vi "Stop Core.vi"(10 "final error code":i32, 11 "CONTADOR_CON_LIMITES in":refnum<class "CONTADOR_CON_LIMITES.lvclass">) -> (3 "CONTADOR_CON_LIMITES out":refnum<class "CONTADOR_CON_LIMITES.lvclass">)   [LabVIEW 2019, in "CONTADOR_CON_LIMITES.lvlib" / "CONTADOR_CON_LIMITES.lvclass"]
doc: "(<B>Filename</B>: Actor Framework.lvlib:Actor.lvclass:Stop Core.vi)\n\nDefines what the actor does before it stops. Use the <B>final error code</B> input to determine whether the actor shut down in response to an error.\n\nBy default, this method passes the Stop message along to all auto-stop nested actors. A descendant class may override this method to define additional behavior, such as shutting down any processes the actor initiated in its override of the Actor Core method."
uses:
  CONTADOR_CON_LIMITES.lvclass
  <vilib>/ActorFramework/Actor/Actor.lvclass
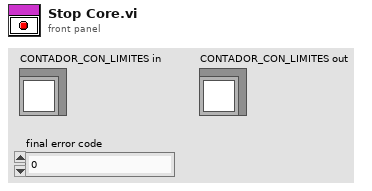
[diagram p1: front panel]
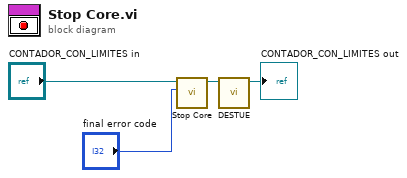
[diagram p0: block diagram]
diagram:
  n1 = call-parent "Stop Core.vi"("final error code"="final error code", "Actor in"="CONTADOR_CON_LIMITES in") -> ("Actor out"=w2:refnum<class "CONTADOR_CON_LIMITES.lvclass">)  [unwired: 9 in]
  n2 = call "DESTUE.vi"("CONTADOR_CON_LIMITES in"=w2) -> ("CONTADOR_CON_LIMITES out"=→"CONTADOR_CON_LIMITES out":refnum<class "CONTADOR_CON_LIMITES.lvclass">)  [unwired: 9 in, 1 out]
